vi "Connect.vi"(8 "error in (no error)":errorcluster, 11 "34401 in":refnum<class "34401.lvclass">) -> (0 "error out":errorcluster, 3 "34401 out":refnum<class "34401.lvclass">)   [LabVIEW 2018, in "34401.lvlib" / "34401.lvclass"]
uses:
  34401.lvclass
  34401.lvclass/34401.ctl
  <instrlib>/Agilent 34401/Agilent 34401.lvlib
  PPLs/DMM/Parent/DMM.lvlibp/DMM.lvclass
  C:/Projects/LabVIEW/PPLs/DMM/Parent/DMM.lvlibp/DMM.lvclass
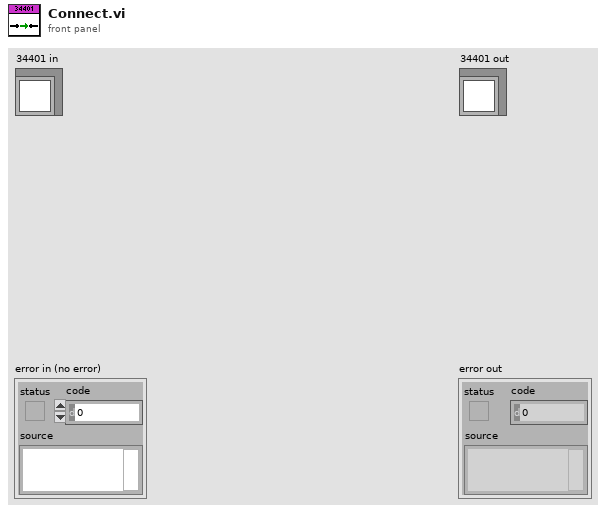
[diagram p1: front panel]
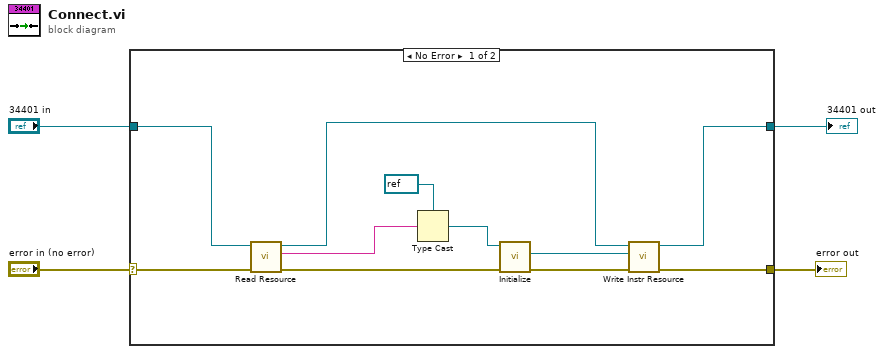
[diagram p0: block diagram]
diagram:
  n1 = case shown="No Error" "error in (no error)" {
    selector: "error in (no error)" -> [w10 w16]
    tunnel: "34401 in" -> [w15 w17]
    tunnel: [w5 w17] -> w3
    tunnel: [w6 w16] -> w1
    frame No Error {
      n2 = call "Read Resource.vi"("error in (no error)"=w10, "DMM in"=w15) -> ("error out"=w11:errorcluster, "Resource"=w14:string, "DMM out"=w9:refnum<class "34401.lvclass">)  [unwired: 7 in]
      n3 = Type Cast(type=refnum<visa-resource-name> refnum ("VISA resource name"), x=w14) -> (*(type *) &x=w12:refnum<visa-resource-name>)
      n4 = call <instrlib>:"Initialize.vi"("error in (no error)"=w11, "VISA resource name"=w12) -> ("error out"=w7:errorcluster, "VISA resource name out"=w8:refnum<visa-resource-name>)  [unwired: 8 in]
      n5 = call "Write Instr Resource.vi"("error in (no error)"=w7, "Instr Resource"=w8, "34401 in"=w9) -> ("error out"=w6:errorcluster, "34401 out"=w5:refnum<class "34401.lvclass">)  [unwired: 7 in]
    }
    frame Error {
    }
  }
  "error out" <- w1
  "34401 out" <- w3
